vi "AnaliseOnline.vi"() -> ()   [LabVIEW 2014, in "Aquisicao de Dados.lvlib"]
uses:
  Aquisicao de Dados.lvlib
panel:
  out "Waveform Graph":waveform(dbl)[](graph)
  in  "stop":bool
  in  "Método de Entrada":T1(ring)
  in  "Amostras por Iteração":i32=2000
  out "Error Out":errorcluster
  in  "Error In":errorcluster
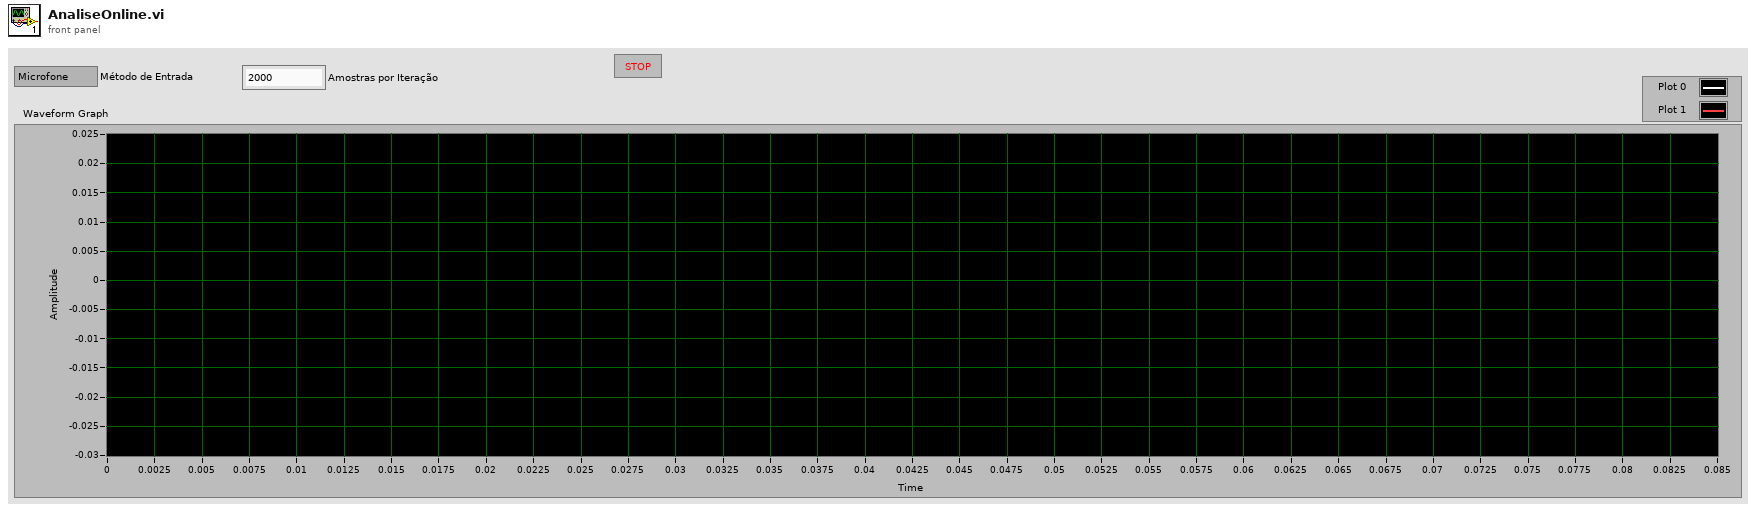
[diagram p1: front panel]
types:
  T1 = enum16{"Microfone", "Arduino", "LTSpice", "Arquivo WAV"}
  T2 = typedef "Aquisicao de Dados.lvlib/_ACC_DATA_ Config DAta State.ctl" = cluster{"_RAW_ Traces":cluster{"Trace Name":string, "Trace Type":string, "Trace Raw Data":dbl[], "Trace Waveform":waveform(dbl)}[], "_WAV_ Traces":waveform(dbl)[], "_MIC_ Config":cluster{"task ID":T3, "Data Chunk Size":i32, "Num Channels":i32, "Resolution":i32, "Sampling Frequency":dbl, "device ID":u32, "Num Chunks":i32}, "_LVM_ Traces":cluster{"Trace Name":string, "Trace Type":string, "Trace Raw Data":dbl[], "Trace Waveform":waveform(dbl)}[]}
  T3 = typedef "Sound Input Task ID.ctl" = u32
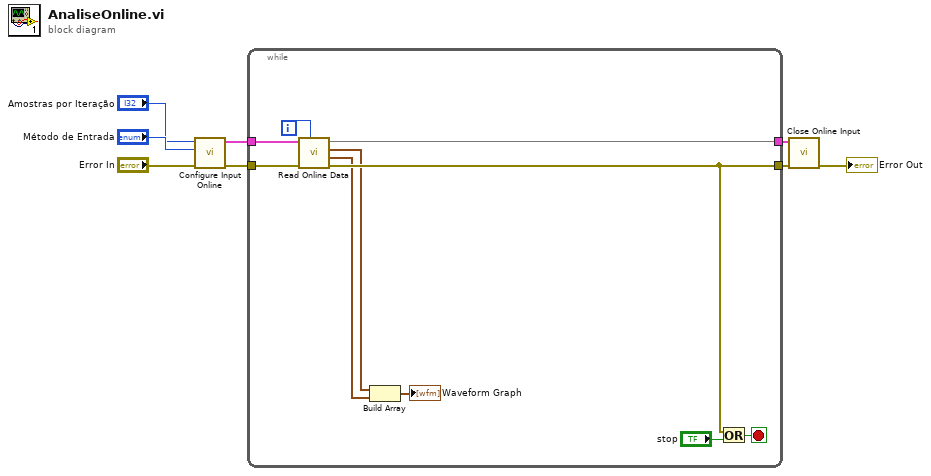
[diagram p0: block diagram]
diagram:
  n1 = call "Configure Input Online.vi"("Error In"="Error In", 10:"Método de Entrada", 11:"Amostras por Iteração") -> ("Error Out"=w4:errorcluster, "Config Out"=w1:T2)  [unwired: 6 in, 1 out]
  n2 = while {
    tunnel: w4 -> [w18]
    tunnel: [w12] -> w3
    tunnel: [w15] -> w2
    tunnel: w1 -> [w17]
    i -> [w16]
    stop <- w14 stop-if-true
    n3 = call "Read Online Data.vi"(7:w16, "Error In"=w18, "Config Out"=w17) -> ("Error Out"=w12:errorcluster, "Channel 1"=w11:waveform(dbl), "Channel 0"=w9:waveform(dbl), 3:w15)  [unwired: 5 in]
    n4 = Build Array(w9, w11) -> (→"Waveform Graph":waveform(dbl)[])
    n5 = Or(x=w12, y="stop") -> (x .or. y?=w14:bool)
  }
  n6 = call "Close Online Input.vi"("Error In"=w3, "Config In"=w2) -> ("Error Out"=→"Error Out":errorcluster)  [unwired: 9 in]
